vi "Execution_Message_Act.vi"(7 "EVE reference in":refnum<data-value>, 8 "error in (no error)":errorcluster, 11 "Messages in":refnum<class "Messages.lvclass">) -> (0 "error out":errorcluster, 3 "Messages out":refnum<class "Messages.lvclass">)   [LabVIEW 2013, in "Messages.lvclass"]
uses:
  Messages.lvclass
  EVE/EVE.lvclass
  100_PROCESS/Class/Process/EnumProcess.ctl
  100_PROCESS/Class/Process/Process.lvclass
  100_PROCESS/01_MessageHandlerProcess/Class/MessageHandler.lvclass
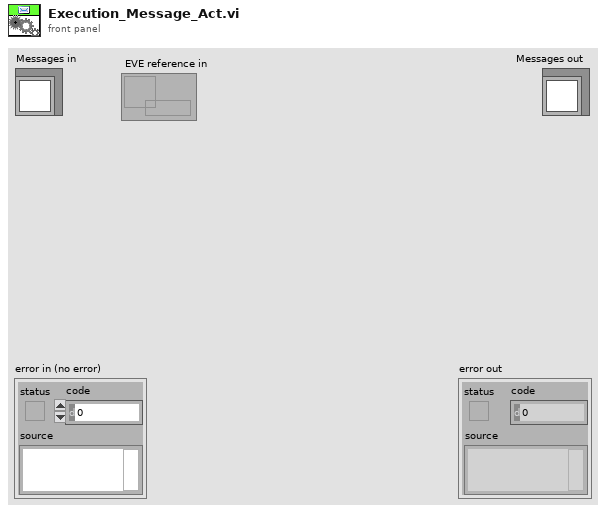
[diagram p1: front panel]
types:
  T1 = typedef "Process.lvclass/EnumProcess.ctl" = enum16{"Message handler", "Template"}
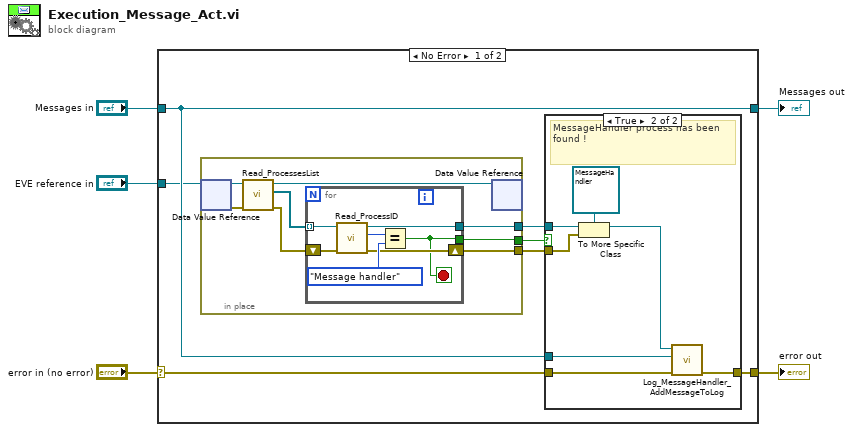
[diagram p0: block diagram]
diagram:
  n1 = case shown="No Error" "error in (no error)" {
    selector: "error in (no error)" -> [w12 w37]
    tunnel: [w11 w37] -> w4
    tunnel: [w10 w36] -> w2
    tunnel: "Messages in" -> [w10 w36]
    tunnel: "EVE reference in" -> [w9 _]
    frame No Error {
      n2 = in-place {
        in-place-border: [w23] -> w8
        in-place-border: [w22] -> w7
        in-place-border: [w21] -> w6
        n3 = in-place-dvr #1(w9) -> (w28:refnum<class "EVE.lvclass">, w27:errorcluster)
        n4 = call-dynamic "Read_ProcessesList.vi"("error in (no error)"=w27, "EVE in"=w28) -> ("error out"=w24:errorcluster, "List"=w26:refnum<class "Process.lvclass">[], "EVE out"=w25:refnum<class "EVE.lvclass">)  [unwired: 7 in]
        n5 = for {
          tunnel: w26 -> [w35] mode=indexing
          tunnel: [w31] -> w23
          shift-right: [w30] -> w22
          shift-left: w24 -> [w34]
          tunnel: [w29] -> w21
          stop <- w29 stop-if-true
          n6 = call-dynamic "Read_ProcessID.vi"("error in (no error)"=w34, "Process in"=w35) -> ("error out"=w30:errorcluster, "Process"=w33:T1, "Process out"=w31:refnum<class "Process.lvclass">)  [unwired: 7 in]
          n7 = Equal?(x=w33, y=EnumProcess."Message handler") -> (x = y?=w29:bool)
        }
        n8 = in-place-dvr #1(w25) -> ()  [unwired: 2 out]
      }
      n9 = case shown="True" w6 {
        tunnel: w12 -> [w13 w20]
        tunnel: [w13 w19] -> w11
        tunnel: w10 -> [_ w18]
        tunnel: w8 -> [_ w17]
        tunnel: w7 -> [_ w14]
        frame False {
          # "MessageHandler process has not been found !"
        }
        frame True {
          # "MessageHandler process has been found !"
          n10 = To More Specific Class(target class=refnum<class "MessageHandler.lvclass"> refnum ("MessageHandler.lvclass in"), reference=w17, error in=w14) -> (specific class reference=w15:refnum<class "MessageHandler.lvclass">)  [unwired: 1 out]
          n11 = call "Log_MessageHandler_AddMessageToLog.vi"("error in (no error)"=w20, "Messages.lvclass"=w18, "MessageHandler.lvclass in"=w15) -> ("error out"=w19:errorcluster)  [unwired: 7 in, 1 out]
        }
      }
    }
    frame Error {
    }
  }
  "error out" <- w4
  "Messages out" <- w2
